vi "ParseJSONBody.vi"(8 "error in (no error)":errorcluster, 11 "JSON object in":string) -> (0 "error out":errorcluster, 2 "JSON Error Strings":string[](array[string]), 3 "JSON Response Strings":string[](array[string]))   [LabVIEW 2013]
uses:
  <vilib>/Utility/error.llb/Error Cluster From Error Code.vi
  <vilib>/regexp/Match Regular Expression.xnode
  <vilib>/ErrorRing/Error Ring.xnode
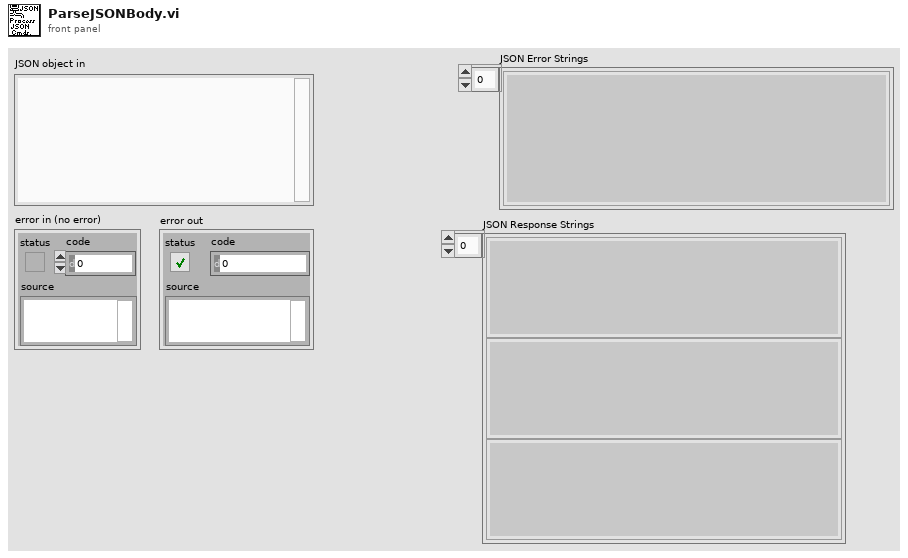
[diagram p1: front panel]
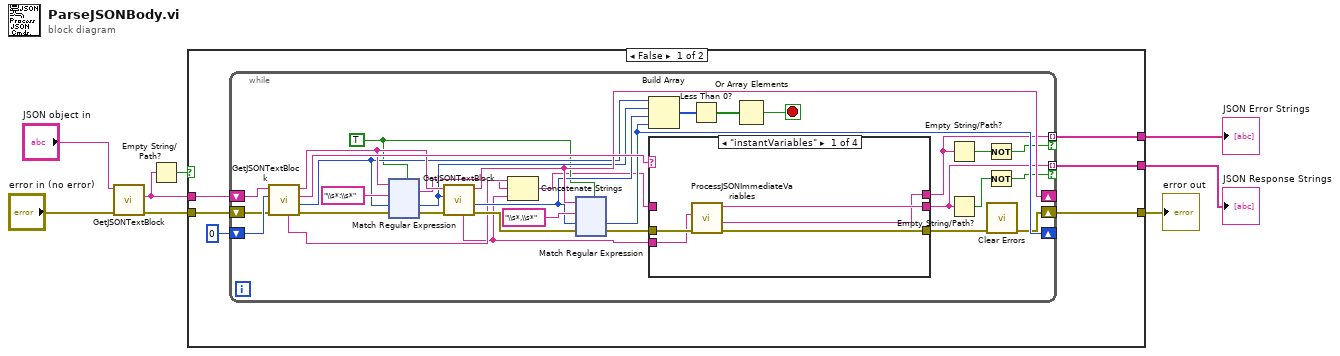
[diagram p0: block diagram]
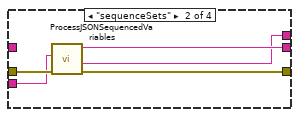
[diagram p2: hidden frame]
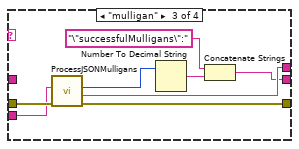
[diagram p3: hidden frame]
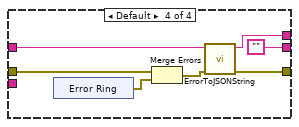
[diagram p4: hidden frame]
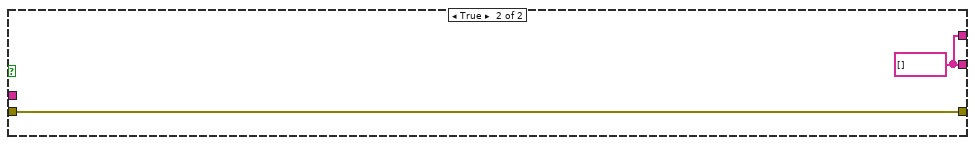
[diagram p5: hidden frame]
diagram:
  n1 = call "GetJSONTextBlock.vi"("error in (no error)"="error in (no error)", "String In"="JSON object in") -> ("error out"=w6:errorcluster, "Matched Block Contents"=w2:string)  [unwired: 5 in, 3 out]
  n2 = Empty String/Path?(string/path=w2) -> (empty?=w1:bool)
  n3 = case shown="False" w1 {
    tunnel: w6 -> [w13 w305]
    tunnel: [w12 w305] -> w5
    tunnel: [w11 w304] -> w4
    tunnel: [w10 w304] -> w3
    tunnel: w2 -> [w9 _]
    frame False {
      n4 = while {
        shift-right: [w36] -> _
        shift-left: w9 -> [w45]
        shift-right: [w32] -> _
        shift-left: 0 -> [w46]
        shift-right: [w15] -> w12
        shift-left: w13 -> [w44]
        tunnel: [w24] -> w11 mode=indexing if=w26
        tunnel: [w18] -> w10 mode=indexing if=w17
        stop <- w30 stop-if-true
        w28 = TRUE ("multiline? (F)")
        n5 = call "GetJSONTextBlock.vi"("error in (no error)"=w44, "Block Start Offset"=w46, "String In"=w45) -> ("error out"=w40:errorcluster, "Offset Past Block"=w35:i32, "Matched Block Contents"=w43:string, "String Out"=w37:string, "Matched Block"=w23:string)  [unwired: 4 in]
        n6 = xnode "Match Regular Expression"("input string"=w37, "regular expression"="\\s*:\\s*", "offset (0)"=w35, "error in"=w40, "multiline? (F)"=w28) -> ("whole match"=w22:string, "offset past match"=w34:i32, "error out"=w39:errorcluster)  [unwired: 1 in, 2 out]
        n7 = call "GetJSONTextBlock.vi"("error in (no error)"=w39, "Block Start Offset"=w34, "String In"=w37) -> ("error out"=w38:errorcluster, "Offset Past Block"=w33:i32, "String Out"=w36:string, "Matched Block"=w21:string)  [unwired: 4 in, 1 out]
        n8 = Concatenate Strings(w23, w22, w21) -> (w20:string)
        n9 = xnode "Match Regular Expression"("input string"=w36, "regular expression"="\\s*,\\s*", "offset (0)"=w33, "error in"=w38, "multiline? (F)"=w28) -> ("offset past match"=w32:i32, "error out"=w27:errorcluster)  [unwired: 1 in, 3 out]
        n10 = Build Array(w35, w34, w33, w32) -> (w31:i32[])
        n11 = case shown="\"instantVariables\"" w43 {
          tunnel: w21 -> [w278 w283 w290 _]
          tunnel: w27 -> [w279 w284 w292 w298]
          tunnel: [w277 w282 w291 w296] -> w16
          tunnel: [w275 w280 w289 w297] -> w24
          tunnel: w20 -> [_ _ _ w294]
          tunnel: [w276 w281 w286 ""] -> w18
          frame "instantVariables" {
            n12 = call "ProcessJSONImmediateVariables.vi"("error in (no error)"=w279, "JSON Array"=w278) -> ("error out"=w277:errorcluster, "JSON Error string"=w275:string, "JSON Response String"=w276:string)  [unwired: 6 in, 1 out]
          }
          frame "sequenceSets" {
            n13 = call "ProcessJSONSequencedVariables.vi"("error in (no error)"=w284, "JSON Array"=w283) -> ("error out"=w282:errorcluster, "JSON Error string"=w280:string, "JSON Response String"=w281:string)  [unwired: 7 in]
          }
          frame "mulligan" {
            n14 = call "ProcessJSONMulligans.vi"("error in (no error)"=w292, "JSON Array"=w290) -> ("error out"=w291:errorcluster, "JSON Error string"=w289:string, "Mulligans Requested"=w288:i32)  [unwired: 7 in]
            n15 = Number To Decimal String(number=w288) -> (decimal integer string=w287:string)  [unwired: 1 in]
            n16 = Concatenate Strings("\"successfulMulligans\":" ("string"), w287) -> (w286:string)
          }
          frame Default {
            n17 = xnode "Error Ring"() -> ("error out"=w299:errorcluster)
            n18 = Merge Errors(w298, w299) -> (w295:errorcluster)
            n19 = call "ErrorToJSONString.vi"("error in (no error)"=w295, "problemJSON"=w294) -> ("error out"=w296:errorcluster, "JSON Error string"=w297:string)  [unwired: 8 in]
          }
        }
        n20 = Less Than 0?(x=w31) -> (x < 0?=w29:bool[])
        n21 = Or Array Elements(Boolean array=w29) -> (logical OR=w30:bool)
        n22 = Empty String/Path?(string/path=w24) -> (empty?=w25:bool)
        n23 = Empty String/Path?(string/path=w18) -> (empty?=w19:bool)
        n24 = Not(x=w25) -> (.not. x?=w26:bool)
        n25 = Not(x=w19) -> (.not. x?=w17:bool)
        n26 = call <vilib>:"Clear Errors.vi"("error in (no error)"=w16) -> ("error out"=w15:errorcluster)  [unwired: 6 in]
      }
    }
    frame True {
      w304 = string[] []
    }
  }
  "error out" <- w5
  "JSON Error Strings" <- w4
  "JSON Response Strings" <- w3
